vi "Perform Action.vi"(8 "error in (no error)":errorcluster, 10 "Input":variant, 11 "DIO DAQmx PWM Fixed Freq CFG in":refnum<class "CO DAQmx Fixed Freq PWM CFG.lvclass">) -> (0 "error out":errorcluster, 2 "Output":variant, 3 "DIO DAQmx PWM Fixed Freq CFG out":refnum<class "CO DAQmx Fixed Freq PWM CFG.lvclass">)   [LabVIEW 2023, in "DAQmx Simulated CFGs.lvlib" / "CO DAQmx Fixed Freq PWM CFG.lvclass"]
uses:
  CO DAQmx Fixed Freq PWM CFG.lvclass
  CO DAQmx Fixed Freq PWM CFG.lvclass/CO DAQmx Fixed Freq PWM CFG.ctl
  DAQmx/DAQmx Base CFG/DAQmx Base CFG.lvclass
panel:
  out "Duty Cycle":dbl
  out "resulting string":string
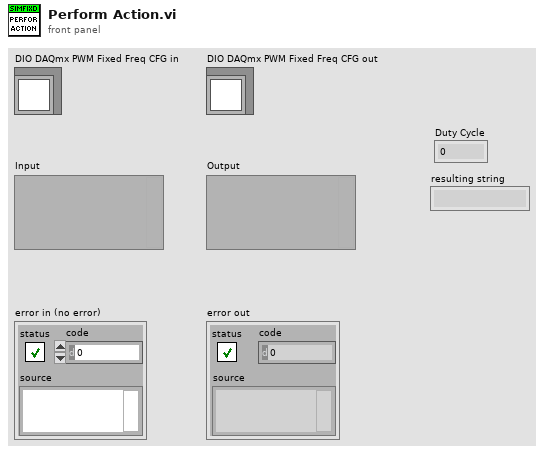
[diagram p1: front panel]
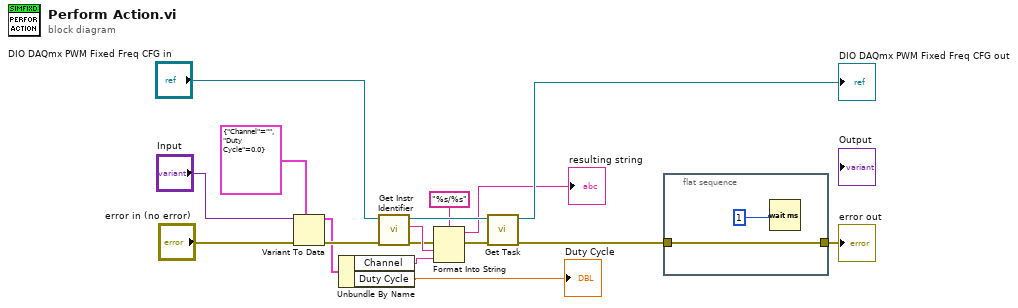
[diagram p0: block diagram]
diagram:
  n1 = Variant To Data(error in="error in (no error)", type=cluster{"Channel":string, "Duty Cycle":dbl} {"Channel"="", "Duty Cycle"=0.0}, Variant="Input") -> (data=w4:cluster{"Channel":string, "Duty Cycle":dbl}, error out=w16:errorcluster)
  n2 = Unbundle By Name(w4) -> ("Channel"=w3:string, "Duty Cycle"=→"Duty Cycle":dbl)
  n3 = call-dynamic "Get Instr Identifier.vi"("error in (no error)"=w16, "Configuration Base in"="DIO DAQmx PWM Fixed Freq CFG in") -> ("error out"=w12:errorcluster, "Instr Ident"=w13:string, "Configuration Base out"=w15:refnum<class "CO DAQmx Fixed Freq PWM CFG.lvclass">)  [unwired: 7 in]
  n4 = Format Into String(format string="%s/%s", error in=w12, w13, w3) -> (resulting string=→"resulting string":string, error out=w1:errorcluster)  [unwired: 1 in]
  n5 = call "Get Task.vi"("DAQmx Base CFG in"=w15) -> ("DAQmx Base CFG out"=→"DIO DAQmx PWM Fixed Freq CFG out":refnum<class "CO DAQmx Fixed Freq PWM CFG.lvclass">)  [unwired: 9 in, 1 out]
  n6 = flat-sequence {
    tunnel: w1 -> [w18]
    tunnel: [w18] -> w6
    frame #0 {
      n7 = Wait (ms)(milliseconds to wait=u32 1) -> ()  [unwired: 1 out]
    }
  }
  "error out" <- w6
